vi "CSDB_Config.get InstanceID.vi"(2 "InstanceName":string, 5 "error in (no error)":errorcluster) -> (16 "InstanceID":string, 17 "entry exists?":bool, 19 "error out":errorcluster)   [LabVIEW 2014, in "CSDB_Config.lvlib"]
doc: "Gets the instance ID of an instance (object)."
uses:
  CSDB_Config.lvlib
  <vilib>/addons/database/_DB Variant To Data/Database Variant To Data.xnode
  <vilib>/addons/database/NI_Database_API.lvlib
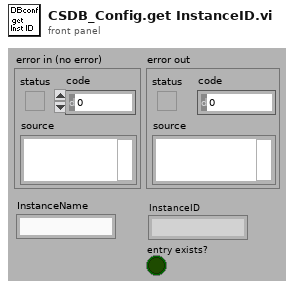
[diagram p1: front panel]
types:
  T1 = typedef "NI_Database_API.lvlib/Conn ObjectReference.ctl" = refnum<k1>
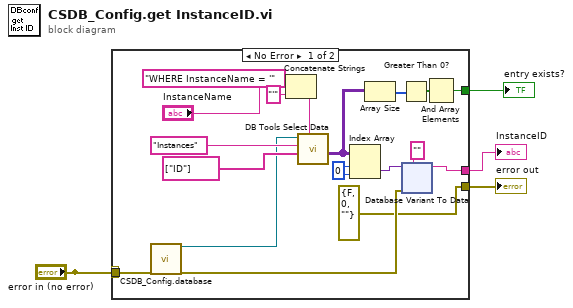
[diagram p0: block diagram]
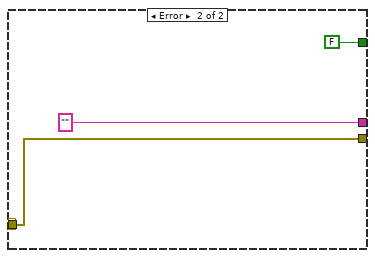
[diagram p2: hidden frame]
diagram:
  n1 = case shown="No Error" "error in (no error)" {
    tunnel: "error in (no error)" -> [w22 w57]
    tunnel: [errorcluster {"status"=FALSE, "code"=0, "source"=""} ("error in (no error)") w57] -> w4
    tunnel: [w11 ""] -> w3
    tunnel: [w7 FALSE] -> w1
    frame No Error {
      w15 = 0 ("index (row)")
      n2 = call "CSDB_Config.database.vi"("error in (no error)"=w22) -> ("connectionRef out"=w5:T1, "error out"=w12:errorcluster)  [unwired: 17 in]
      n3 = Concatenate Strings("WHERE InstanceName = '" ("optional clause"), "InstanceName", "'" ("string")) -> (w16:string)
      n4 = call <vilib>:"DB Tools Select Data.vi"("condition"=w16, "columns"=string[] ["ID"], "table"="Instances", "connection reference"=w5) -> ("data"=w10:variant[][])  [unwired: 2 in, 2 out]
      n5 = Index Array(array=w10, index (row)=w15, index (col)=w15) -> (element=w14:variant)
      n6 = Array Size(array=w10) -> (size(s)=w9:i32[])
      n7 = Greater Than 0?(x=w9) -> (x > 0?=w8:bool[])
      n8 = xnode "Database Variant To Data"("database variant"=w14, "error in (no error)"=w12, "type"="") -> ("data"=w11:string)  [unwired: 1 out]
      n9 = And Array Elements(Boolean array=w8) -> (logical AND=w7:bool)
    }
    frame Error {
    }
  }
  "error out" <- w4
  "InstanceID" <- w3
  "entry exists?" <- w1
